vi "DELETE Y Constant.vi"   [LabVIEW 2013]
uses:
  Action.ctl
  Calibration Output FGV Selector.ctl
types:
  T1 = typedef "Calibration Output FGV Selector.ctl" = enum16{"X Constant", "Y Constant", "Z Constant", "Power Peak", "Slope", "Spring Constant"}
  T2 = typedef "Action.ctl" = enum16{"GET", "PUT", "DELETE"}
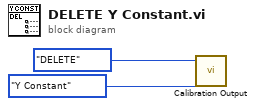
[diagram p0: block diagram]
diagram:
  n1 = call "Calibration Output.vi"("Calibration Output FGV Selector"=Calibration_Output_FGV_Selector."Y Constant", "Action"=Action."DELETE") -> ()  [unwired: 1 in, 1 out]
